vi "Read Light Stack.vi"(8 "error in (no error)":errorcluster, 11 "DigitalIO in":refnum<class "DigitalIO.lvclass">) -> (0 "error out":errorcluster, 2 "Light Stack":refnum<class "Light Stack.lvclass">, 3 "DigitalIO out":refnum<class "DigitalIO.lvclass">)   [LabVIEW 2018, in "DigitalIO.lvlib" / "DigitalIO.lvclass"]
uses:
  DigitalIO.lvclass
  PPLs/PLC/Light Stack.lvlibp/Light Stack.lvclass
  DigitalIO.lvclass/DigitalIO.ctl
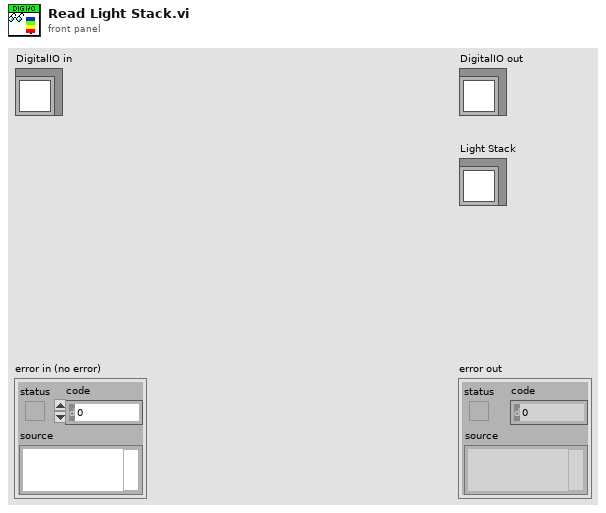
[diagram p1: front panel]
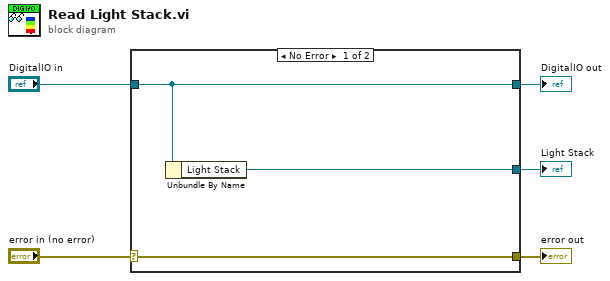
[diagram p0: block diagram]
diagram:
  n1 = case shown="No Error" "error in (no error)" {
    selector: "error in (no error)" -> [w8 w9]
    tunnel: [w8 w9] -> w4
    tunnel: [w7 w10] -> w2
    tunnel: "DigitalIO in" -> [w7 w10]
    tunnel: [w6 _] -> w1
    frame No Error {
      n2 = Unbundle By Name(w7) -> ("Light Stack"=w6:refnum<class "Light Stack.lvclass">)
    }
    frame Error {
    }
  }
  "error out" <- w4
  "DigitalIO out" <- w2
  "Light Stack" <- w1
